vi "1st or last shot of scan.vi"(11 "Command":string) -> (3 "Status":T1)   [LabVIEW 2020, in "Point Grey Camera.lvclass"]
uses:
  Point Grey Camera.lvclass
  1st or last shot of scan.ctl
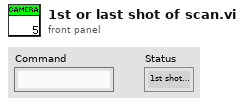
[diagram p1: front panel]
types:
  T1 = typedef "1st or last shot of scan.ctl" = enum16{"1st shot of scan", "1st shot after scan end", "other"}
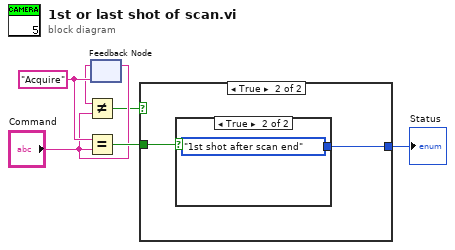
[diagram p0: block diagram]
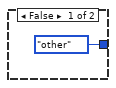
[diagram p2: hidden frame]
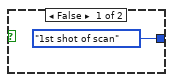
[diagram p3: hidden frame]
diagram:
  w5 = "Acquire" ("Status")
  n1 = Equal?(x=w5, y="Command") -> (x = y?=w6:bool)
  n2 = feedback #1(w5) -> (w1:string)
  n3 = Not Equal?(x=w1, y="Command") -> (x != y?=w2:bool)
  n4 = feedback-in #1("Command") -> ()
  n5 = case shown="True" w2 {
    tunnel: [1st_or_last_shot_of_scan."other" ("Status") w8] -> w3
    tunnel: w6 -> [_ w9]
    frame False {
    }
    frame True {
      n6 = case shown="True" w9 {
        tunnel: [1st_or_last_shot_of_scan."1st shot of scan" ("Status") 1st_or_last_shot_of_scan."1st shot after scan end" ("Status")] -> w8
        frame False {
        }
        frame True {
        }
      }
    }
  }
  "Status" <- w3
